vi "CHS_SIM_Motor_Write.vi"(10 "Motor Demand":dbl, 11 "Motor Device Reference":T1={"DeviceStatus"={"status"=FALSE, "code"=0, "source"=""}, "Type"=enum."PWM", "PWM"={"PWM Channel"=enum."Invalid", "DeadBand"={"Name"="", "maxPositivePwm"=0, "minPositivePwm"=0, "centerPwm"=0, "maxNegativePwm"=0, "minNegativePwm"=0, "angularRange"=0}}, "CAN"={"Device Number"=0, "SetOutput VI Ref"=variant, "GetOutput VI Ref"=variant, "Enable VI Ref"=variant, "Disable VI Ref"=variant, "Data"=variant}, "Invert"=FALSE, "DIO PWM"={"PWM \"Enable\" Channel"=enum."Invalid", "DIOChannel"=enum."Invalid", "PWM Rate"=0.0}}) -> (3 "Out Motor Demand":dbl)   [LabVIEW 2019]
uses:
  CHS_SIM_SIM_Globals.vi
  <vilib>/Rock Robotics/WPI/ThirdParty/JAS_Junk/TrajLib/Trajectory_Library.lvlib
  <vilib>/Rock Robotics/SystemInterfaces/DIO/FPGA_DIOPWMChannel.ctl
  <vilib>/Rock Robotics/WPI/PWM/WPI_PWMDeadband.ctl
  <vilib>/Rock Robotics/WPI/MotorControl/WPI_MotorControlType.ctl
  <vilib>/Rock Robotics/SystemInterfaces/DIO/FPGA_DIOChannel.ctl
  <vilib>/Rock Robotics/WPI/MotorControl/WPI_MotorControlDeviceRef.ctl
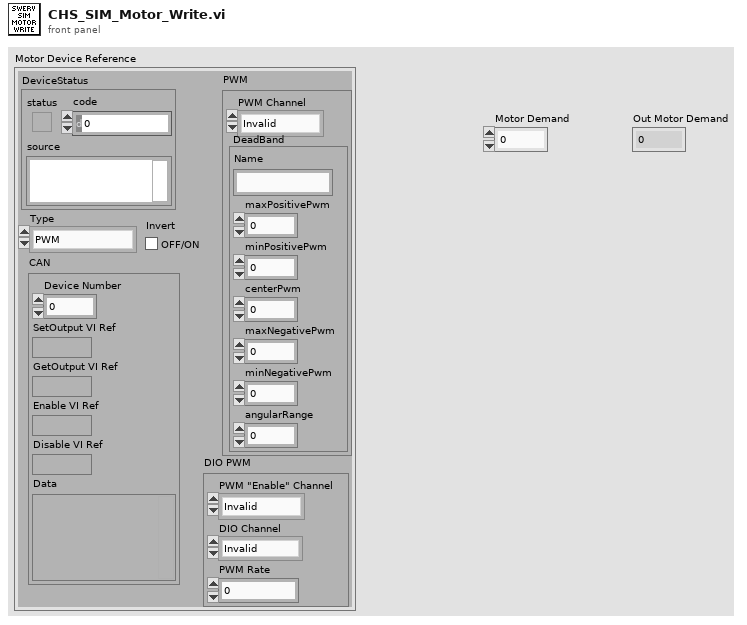
[diagram p1: front panel]
types:
  T1 = typedef "WPI_MotorControlDeviceRef.ctl" = cluster{"DeviceStatus":errorcluster, "Type":T2, "PWM":cluster{"PWM Channel":T3, "DeadBand":T4}, "CAN":cluster{"Device Number":u8, "SetOutput VI Ref":variant, "GetOutput VI Ref":variant, "Enable VI Ref":variant, "Disable VI Ref":variant, "Data":variant}, "Invert":bool, "DIO PWM":cluster{"PWM \"Enable\" Channel":T3, "DIOChannel":T5, "PWM Rate":dbl}}
  T2 = typedef "WPI_MotorControlType.ctl" = enum16{"PWM", "CAN", "DIO PWM"}
  T3 = typedef "FPGA_DIOPWMChannel.ctl" = enum8{"PWM 0", "PWM 1", "PWM 2", "PWM 3", "PWM 4", "PWM 5", "PWM 6", "PWM 7", "PWM 8", "PWM 9", "PWM MXP 0", "PWM MXP 1", "PWM MXP 2", "PWM MXP 3", "PWM MXP 4", "PWM MXP 5", "PWM MXP 6", "PWM MXP 7", "PWM MXP 8", "PWM MXP 9", "Invalid"}
  T4 = typedef "WPI_PWMDeadband.ctl" = cluster{"Name":string, "maxPositivePwm":i32, "minPositivePwm":i32, "centerPwm":i32, "maxNegativePwm":i32, "minNegativePwm":i32, "angularRange":u16}
  T5 = typedef "FPGA_DIOChannel.ctl" = enum8{"DIO 0", "DIO 1", "DIO 2", "DIO 3", "DIO 4", "DIO 5", "DIO 6", "DIO 7", "DIO 8", "DIO 9", "DIO MXP 0", "DIO MXP 1", "DIO MXP 2", "DIO MXP 3", "DIO MXP 4", "DIO MXP 5", "DIO MXP 6", "DIO MXP 7", "DIO MXP 8", "DIO MXP 9", "DIO MXP 10", "DIO MXP 11", "DIO MXP 12", "DIO MXP 13", "DIO MXP 14", "DIO MXP 15", "SPI Port CS1", "SPI Port CS2", "SPI Port CS3", "SPI Port MISO", "SPI Port MOSI", "Invalid"}
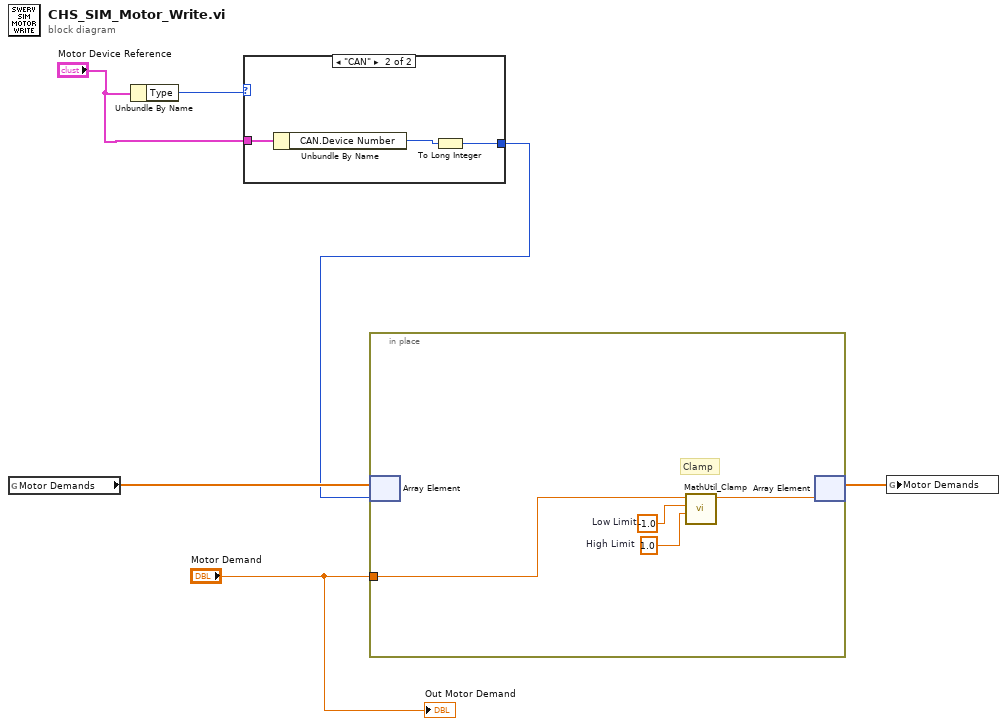
[diagram p0: block diagram]
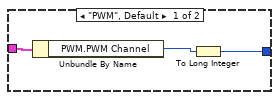
[diagram p2: hidden frame]
diagram:
  n1 = global read "CHS_SIM_SIM_Globals.vi" "Motor Demands"() -> (w6:dbl[])
  n2 = Unbundle By Name("Motor Device Reference") -> ("Type"=w5:T2)
  n3 = case shown="\"CAN\"" w5 {
    tunnel: "Motor Device Reference" -> [w9 w11]
    tunnel: [w7 w10] -> w3
    frame "PWM", Default {
      n4 = Unbundle By Name(w9) -> ("PWM.PWM Channel"=w8:T3)
      n5 = To Long Integer(number=w8) -> (32bit integer=w7:i32)
    }
    frame "CAN" {
      n6 = Unbundle By Name(w11) -> ("CAN.Device Number"=w12:u8)
      n7 = To Long Integer(number=w12) -> (32bit integer=w10:i32)
    }
  }
  n8 = in-place {
    in-place-border: "Motor Demand" -> [w14]
    w16 = 1.0  # High Limit
    w15 = -1.0  # Low Limit
    # "Clamp"
    n9 = in-place-array #1(w6, w3) -> ()  [unwired: 1 out]
    n10 = call <vilib>:"MathUtil_Clamp.vi"("High Limit"=w16, "Low Limit"=w15, "Value"=w14) -> ("Result"=w13:dbl)  [unwired: 8 in]
    n11 = in-place-array #1(w13) -> (w2:dbl[])  [unwired: 1 out]
  }
  n12 = global write "CHS_SIM_SIM_Globals.vi" "Motor Demands"(w2) -> ()
  "Out Motor Demand" <- "Motor Demand"
